vi "Robot arm_labview.vi"() -> ()   [LabVIEW 2022 SP3]
uses:
  <vilib>/MakerHub/LINX/Public/Utilities/Open Serial.vi
  <vilib>/MakerHub/LINX/Public/Sensors/Motion/Servo/Servo Open One Channel.vi
  <vilib>/MakerHub/LINX/Public/Sensors/Motion/Servo/Servo Set Pulse Width One Channel.vi
  <vilib>/MakerHub/LINX/Public/Sensors/Motion/Servo/Servo Close One Channel.vi
  <vilib>/MakerHub/LINX/LMH-LINX.lvlib
  <vilib>/MakerHub/LINX/Public/Sensors/Motion/Servo/Servo.lvlib
  Global 2 Horizontal.vi
  Global 3 Vertical.vi
  Global 4 Arm.vi
panel:
  in  "Arm":bool
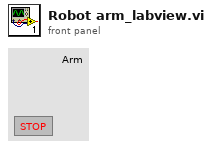
[diagram p1: front panel]
types:
  T1 = typedef "LMH-LINX.lvlib/LINX Ref.ctl" = cluster{"IO":T2, "Interface":T3, "LINX Device Config":T4}
  T2 = typedef "LMH-LINX.lvlib/Platform.ctl" = enum16{"Remote", "Local"}
  T3 = typedef "LMH-LINX.lvlib/Interface.ctl" = enum16{"Serial", "TCP"}
  T4 = typedef "LMH-LINX.lvlib/Device.lvlib/LINX Device Config.ctl" = cluster{"Interface":T3, "COM Port":refnum<visa-resource-name>, "TCP Configuration":T5, "Device Family":u8, "Device ID":u8, "Device Name":string, "TCP Ref":refnum<k5>, "Channels":T6}
  T5 = typedef "LMH-LINX.lvlib/Device.lvlib/TCP Config.ctl" = cluster{"IP Address":string, "Port":u16}
  T6 = typedef "LMH-LINX.lvlib/Channels.ctl" = cluster{"DI":u8[], "DO":u8[], "AI":u8[], "AO":u8[], "PWM":u8[], "QE":u8[], "UART":u8[], "I2C 2":u8[], "SPI":u8[], "CAN":u8[], "Servo":u8[], "AI Ref (V)":dbl, "AI Resolution (Bits)":u8, "AO Ref (V)":dbl, "AO Resolution (Bits)":u8}
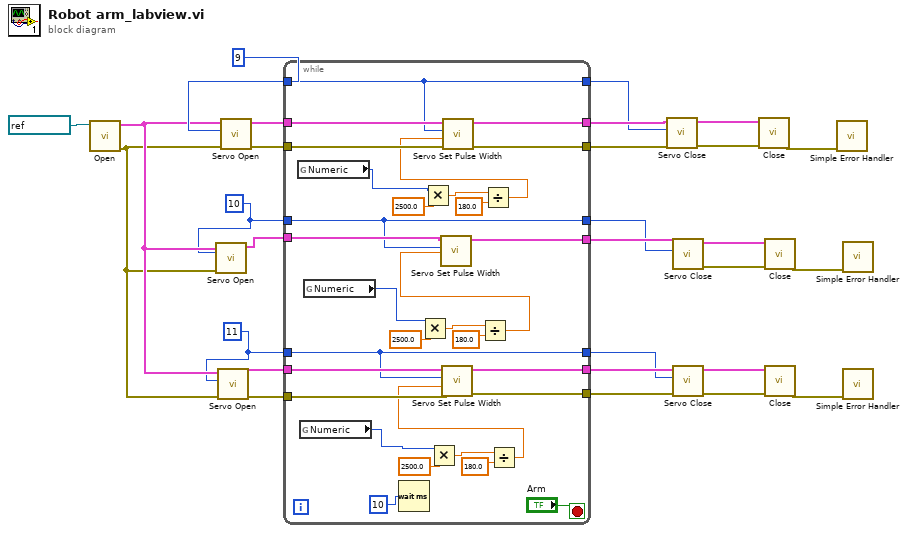
[diagram p0: block diagram]
diagram:
  w5 = 11
  w3 = 10
  w23 = 9
  n1 = call-poly <vilib>:"Open.vi"("Serial Port"=refnum<visa-resource-name> "COM6") -> ("Error Out"=w6:errorcluster, "LINX Resource"=w7:T1)  [unwired: 8 in, 1 out]
  n2 = call-poly <vilib>:"Servo Open.vi"("Error In"=w6, "Servo Channel"=w3, "LINX Resource"=w7) -> ("LINX Resource"=w13:T1)  [unwired: 7 in, 1 out]
  n3 = call-poly <vilib>:"Servo Open.vi"("Error In"=w6, "Servo Channel"=w5, "LINX Resource"=w7) -> ("Error Out"=w9:errorcluster, "LINX Resource"=w10:T1)  [unwired: 7 in]
  n4 = call-poly <vilib>:"Servo Open.vi"("Error In"=w6, "Servo Channel"=w23, "LINX Resource"=w7) -> ("Error Out"=w25:errorcluster, "LINX Resource"=w27:T1)  [unwired: 7 in]
  n5 = while {
    tunnel: w27 -> [w56]
    tunnel: [w55] -> w26
    tunnel: w25 -> [w54]
    tunnel: [w53] -> w24
    tunnel: w23 -> [w44]
    tunnel: w13 -> [w52]
    tunnel: [w51] -> w12
    tunnel: [w50] -> w11
    tunnel: w10 -> [w49]
    tunnel: w9 -> [w48]
    tunnel: [w47] -> w8
    tunnel: w5 -> [w46]
    tunnel: [w46] -> w4
    tunnel: w3 -> [w45]
    tunnel: [w45] -> w2
    tunnel: [w44] -> w1
    stop <- "Arm" stop-if-true
    n6 = global read "Global 2 Horizontal.vi" "Numeric"() -> (w31:i32)
    n7 = global read "Global 4 Arm.vi" "Numeric"() -> (w30:i32)
    n8 = global read "Global 3 Vertical.vi" "Numeric"() -> (w29:i32)
    n9 = Wait (ms)(milliseconds to wait=u32 10) -> ()  [unwired: 1 out]
    n10 = Multiply(x=w29, y=2500.0) -> (x*y=w40:dbl)
    n11 = Multiply(x=w31, y=2500.0) -> (x*y=w43:dbl)
    n12 = Multiply(x=w30, y=2500.0) -> (x*y=w37:dbl)
    n13 = Divide(x=w40, y=180.0) -> (x/y=w33:dbl)
    n14 = call-poly <vilib>:"Servo Set Pulse Width.vi"("Pulse Width (uS)"=w33, "Servo Channel"=w45, "LINX Resource"=w52) -> ("LINX Resource"=w51:T1)  [unwired: 7 in, 1 out]
    n15 = Divide(x=w43, y=180.0) -> (x/y=w32:dbl)
    n16 = call-poly <vilib>:"Servo Set Pulse Width.vi"("Error In"=w54, "Pulse Width (uS)"=w32, "Servo Channel"=w44, "LINX Resource"=w56) -> ("Error Out"=w53:errorcluster, "LINX Resource"=w55:T1)  [unwired: 6 in]
    n17 = Divide(x=w37, y=180.0) -> (x/y=w34:dbl)
    n18 = call-poly <vilib>:"Servo Set Pulse Width.vi"("Error In"=w48, "Pulse Width (uS)"=w34, "Servo Channel"=w46, "LINX Resource"=w49) -> ("Error Out"=w47:errorcluster, "LINX Resource"=w50:T1)  [unwired: 6 in]
  }
  n19 = call-poly <vilib>:"Servo Close.vi"("Error In"=w24, "Servo Channel"=w1, "LINX Resource"=w26) -> ("Error Out"=w20:errorcluster, "LINX Resource"=w21:T1)  [unwired: 7 in]
  n20 = call-poly <vilib>:"Servo Close.vi"("Servo Channel"=w2, "LINX Resource"=w12) -> ("Error Out"=w17:errorcluster, "LINX Resource"=w18:T1)  [unwired: 8 in]
  n21 = call-poly <vilib>:"Servo Close.vi"("Error In"=w8, "Servo Channel"=w4, "LINX Resource"=w11) -> ("Error Out"=w14:errorcluster, "LINX Resource"=w15:T1)  [unwired: 7 in]
  n22 = call <vilib>:"Close.vi"("Error In"=w20, "LINX Resource"=w21) -> ("Error Out"=w22:errorcluster)  [unwired: 9 in]
  n23 = call <vilib>:"Close.vi"("Error In"=w17, "LINX Resource"=w18) -> ("Error Out"=w19:errorcluster)  [unwired: 9 in]
  n24 = call <vilib>:"Close.vi"("Error In"=w14, "LINX Resource"=w15) -> ("Error Out"=w16:errorcluster)  [unwired: 9 in]
  n25 = call <vilib>:"Simple Error Handler.vi"("error in (no error)"=w22) -> ()  [unwired: 4 in, 5 out]
  n26 = call <vilib>:"Simple Error Handler.vi"("error in (no error)"=w19) -> ()  [unwired: 4 in, 5 out]
  n27 = call <vilib>:"Simple Error Handler.vi"("error in (no error)"=w16) -> ()  [unwired: 4 in, 5 out]
